vi "gun_reload_conf.vi"() -> ()   [LabVIEW 2011]
panel:
  in  "Cluster":T1
  in  "Do Reload Conf":bool
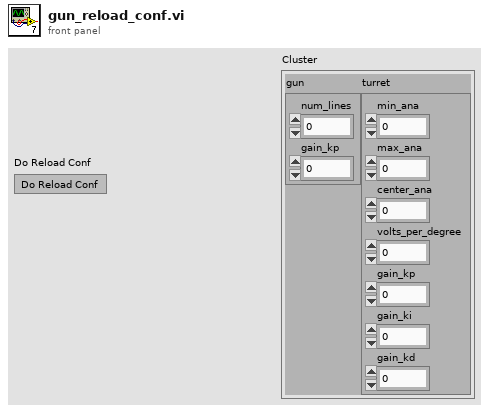
[diagram p1: front panel]
types:
  T1 = cluster{"gun":cluster{"num_lines":dbl, "gain_kp":dbl}, "turret":cluster{"min_ana":dbl, "max_ana":dbl, "center_ana":dbl, "volts_per_degree":dbl, "gain_kp":dbl, "gain_ki":dbl, "gain_kd":dbl}}
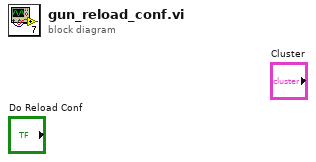
[diagram p0: block diagram]
diagram:
